vi "GUNSC_LibGetRawPtr.vi"(8 "error in (no error)":errorcluster) -> (0 "error out":errorcluster, 1 "namps":i32, 2 "raw image ptr":u64)   [LabVIEW 2014]
uses:
  public/c/lib/libunsc.so
panel:
  in  "namps ctrl":i32
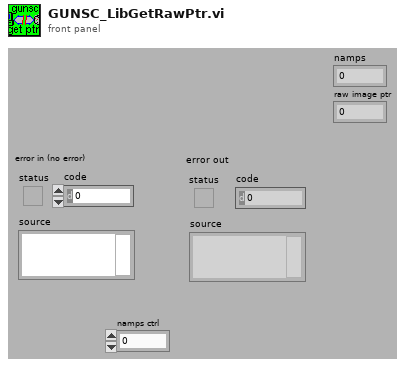
[diagram p1: front panel]
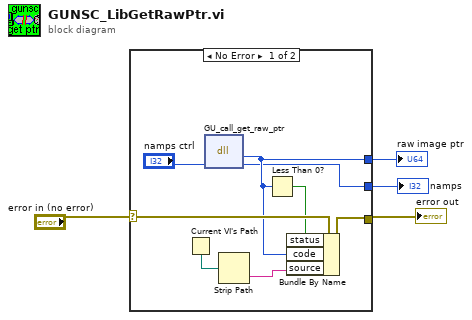
[diagram p0: block diagram]
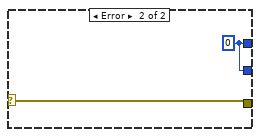
[diagram p2: hidden frame]
diagram:
  n1 = case shown="No Error" "error in (no error)" {
    selector: "error in (no error)" -> [w12 w14]
    tunnel: [w10 w13] -> w4
    tunnel: [w7 w14] -> w2
    tunnel: [w5 w13] -> w1
    frame No Error {
      n2 = Current VI's Path() -> (path=w9:path)
      n3 = dll-call lib="home/sispi/Panview-1.13.0-64b/PAN/Modules/GUNSC/public/c/lib/libunsc.so" fn="GU_call_get_raw_ptr"("namps"="namps ctrl") -> ("return type"=w10:u64, "namps"=w5:i32)  [unwired: 3 in, 2 out]
      n4 = Strip Path(path=w9) -> (name=w8:string)  [unwired: 1 out]
      n5 = Less Than 0?(x=w10) -> (x < 0?=w11:bool)
      n6 = Bundle By Name(cluster=w12, "status"=w11, "code"=w10, "source"=w8) -> (w7:errorcluster)
    }
    frame Error {
      w13 = 0
    }
  }
  "raw image ptr" <- w4
  "error out" <- w2
  "namps" <- w1
